vi "test LoadSeq parsing.vi"() -> ()   [LabVIEW 2017]
uses:
  LV_Source/Subsystems/Sequencer/Sequencer.lvclass
  LV_Source/Subsystems/Sequencer/DataTypes/SeqFileParam_OscMode--enum.ctl
  LV_Source/Subsystems/Sequencer/DataTypes/SeqFileParameters--cluster.ctl
  LV_Source/Subsystems/Sequencer/DataTypes/SeqStep_LockoutState--enum.ctl
  LV_Source/Subsystems/Sequencer/DataTypes/SeqStep_RampingState--enum.ctl
  LV_Source/Subsystems/Sequencer/DataTypes/SeqStep_PositionerDir--enum.ctl
  LV_Source/Subsystems/Sequencer/DataTypes/SeqStep--cluster.ctl
  LV_Source/Subsystems/Sequencer/DataTypes/SeqFileParam_PosMode--enum.ctl
panel:
  out "Sequence Table":string[][](table)
  out "SeqSteps[]":T1[](array[typedef])
  out "text lines out":string[](array[string])
  out "SeqFileParams":T5
  out "error out":errorcluster
  in  "SeqFile":path
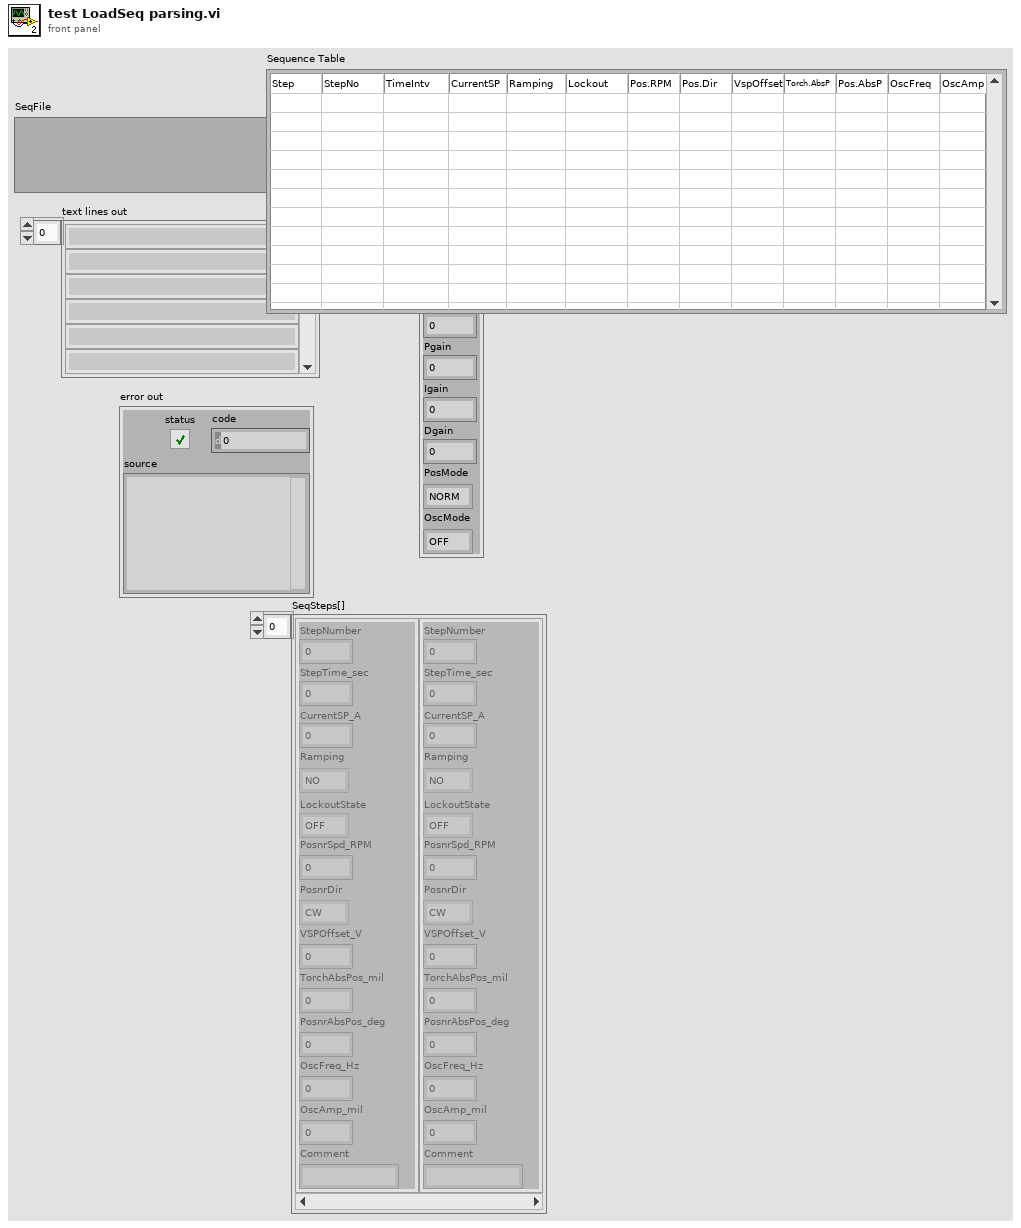
[diagram p1: front panel]
types:
  T1 = typedef "Sequencer.lvclass/SeqStep--cluster.ctl" = cluster{"StepNumber":i32, "StepTime_sec":dbl, "CurrentSP_A":dbl, "Ramping":T2, "LockoutState":T3, "PosnrSpd_RPM":dbl, "PosnrDir":T4, "VSPOffset_V":dbl, "TorchAbsPos_mil":dbl, "PosnrAbsPos_deg":dbl, "OscFreq_Hz":dbl, "OscAmp_mil":dbl, "Comment":string}
  T2 = typedef "Sequencer.lvclass/SeqStep_RampingState--enum.ctl" = enum16{"NO", "YES"}
  T3 = typedef "Sequencer.lvclass/SeqStep_LockoutState--enum.ctl" = enum16{"OFF", "ON"}
  T4 = typedef "Sequencer.lvclass/SeqStep_PositionerDir--enum.ctl" = enum16{"CW", "CCW"}
  T5 = typedef "Sequencer.lvclass/SeqFileParameters--cluster.ctl" = cluster{"MotorVel":dbl, "VoltageSP":dbl, "MoveSF":dbl, "IntegTime":dbl, "Pgain":dbl, "Igain":dbl, "Dgain":dbl, "PosMode":T6, "OscMode":T7}
  T6 = typedef "Sequencer.lvclass/SeqFileParam_PosMode--enum.ctl" = enum16{"NORM", "ABS"}
  T7 = typedef "Sequencer.lvclass/SeqFileParam_OscMode--enum.ctl" = enum16{"OFF", "ON"}
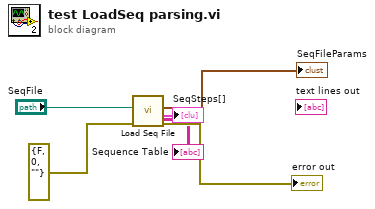
[diagram p0: block diagram]
diagram:
  n1 = call "Load Seq File.vi"("error in (no error)"=errorcluster {"status"=FALSE, "code"=0, "source"=""} ("error in"), "SeqFile"="SeqFile") -> ("error out"=→"error out":errorcluster, "SeqSteps[]"=→"SeqSteps[]":T1[], "SeqFileParams"=→"SeqFileParams":T5, "Sequence Table"=→"Sequence Table":string[][])  [unwired: 4 in, 2 out]
